vi "Copy PDC To VI.vi"(8 "error in (no error)":errorcluster, 10 "LVClassLibrary Refnum in":refnum<vi>, 11 "VI in":refnum<vi>) -> (0 "error out":errorcluster, 1 "LVClassLibrary Refnum out":refnum<vi>, 2 "Cluster Ref":refnum<vi>, 3 "VI out":refnum<vi>)   [LabVIEW 2019, in "gRPC Template Creation Utility.lvlib"]
uses:
  gRPC Template Creation Utility.lvlib
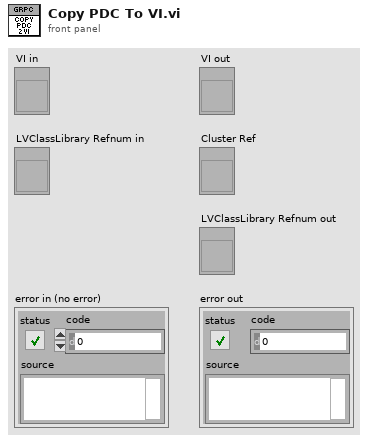
[diagram p1: front panel]
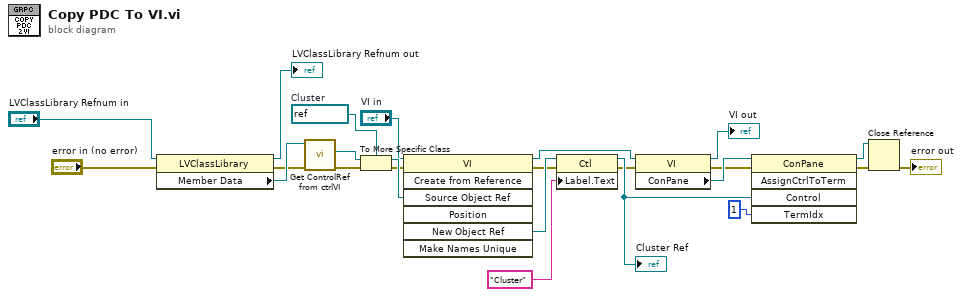
[diagram p0: block diagram]
diagram:
  w20 = refnum<vi> refnum  # Cluster
  n1 = property class="LVClassLibrary"(reference="LVClassLibrary Refnum in", error in="error in (no error)") -> (reference out=→"LVClassLibrary Refnum out":refnum<vi>, error out=w19:errorcluster, "Member Data"=w23:refnum<vi>)
  n2 = call "Get ControlRef from ctrlVI.vi"("error in (no error)"=w19, "VI ref in"=w23) -> ("error out"=w14:errorcluster, "Control ref out"=w21:refnum<vi>)  [unwired: 7 in, 1 out]
  n3 = To More Specific Class(target class=w20, reference=w21, error in=w14) -> (specific class reference=w22:refnum<vi>, error out=w13:errorcluster)
  n4 = invoke class="VI" method="Create from Reference"(reference="VI in", error in=w13, "Source Object Ref"=w22) -> (reference out=w7:refnum<vi>, error out=w11:errorcluster, "New Object Ref"=w24:refnum<vi>)  [unwired: 4 in, 4 out]
  n5 = property class="Ctl"(reference=w24, error in=w11, "Label.Text"="Cluster") -> (reference out=w9:refnum<vi>, error out=w3:errorcluster)
  "Cluster Ref" <- w9
  n6 = property class="VI"(reference=w7, error in=w3) -> (reference out=→"VI out":refnum<vi>, error out=w2:errorcluster, "ConPane"=w10:refnum<vi>)
  n7 = invoke class="ConPane" method="AssignCtrlToTerm"(reference=w10, error in=w2, "Control"=w9, "TermIdx"=u32 1 ("Terminal Index")) -> (reference out=w4:refnum<vi>, error out=w5:errorcluster)  [unwired: 1 in, 3 out]
  n8 = Close Reference(reference=w4, error in (no error)=w5) -> (error out=→"error out":errorcluster)
